vi "Get QE.vi"(7 "QE":sgl, 8 "error in (no error)":errorcluster, 9 "mode":u32, 10 "wavelength":sgl, 11 "sensor":string) -> (0 "error out":errorcluster, 2 "function return":u32, 3 "sensor out":string, 5 "QE out":sgl)   [LabVIEW 2014, in "atmcd32d.lvlib"]
doc: "unsigned int WINAPI GetQE(char * sensor, float wavelength, unsigned int mode, float * QE);"
uses:
  atmcd32d.lvlib
  atmcd32d.dll
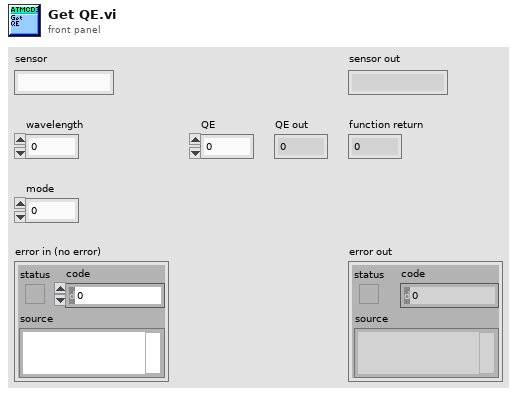
[diagram p1: front panel]
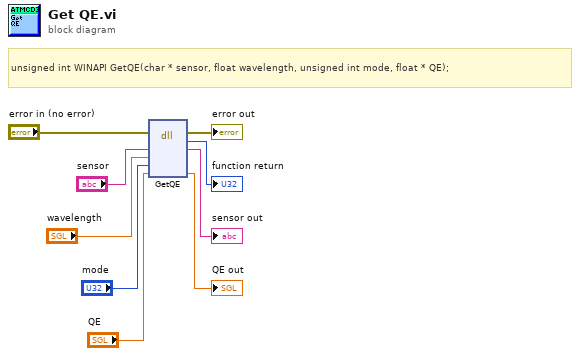
[diagram p0: block diagram]
diagram:
  # "unsigned int WINAPI GetQE(char * sensor, float wavelength, unsigned int mode, float * QE);"
  n1 = dll-call lib="C:/Users/Bakir/Documents/Lambda2-Testing/lib/Andorlib/atmcd32d.*" fn="GetQE"(error in="error in (no error)", "sensor"="sensor", "wavelength"="wavelength", "mode"="mode", "QE"="QE") -> (error out=→"error out":errorcluster, →"function return":u32, "sensor"=→"sensor out":string, "QE"=→"QE out":sgl)  [unwired: 4 in, 1 out]
